vi "Insight_R_Synch_Index.vi"(8 "error in (no error)":errorcluster, 11 "telnet connection":T1) -> (0 "error out":errorcluster, 1 "response data":string, 2 "Index of Synch Pulse":u32, 3 "telnet  connection out":T1)   [LabVIEW 2015]
doc: "Insight Photonic Solutions\n\nThis VI reads the index of the Synchronization Pulse from the Synchronization sweep of the laser. Use this index, in comparison with a detected and acquired pulse, to synchronization the sweep with the acquisition.\n\nver 1.0 - original release\nver 1.1 - added output for the response data buffer"
uses:
  Telnet Session.ctl
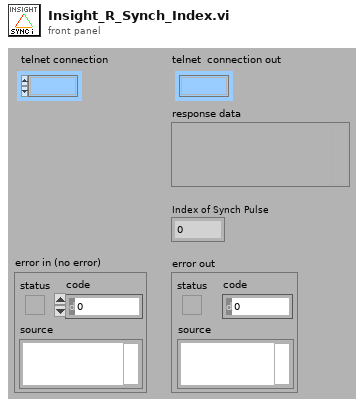
[diagram p1: front panel]
types:
  T1 = typedef "Telnet Session.ctl" = refnum<k1>
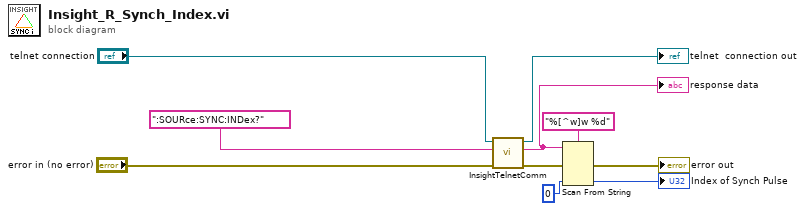
[diagram p0: block diagram]
diagram:
  n1 = call "InsightTelnetComm.vi"("error in"="error in (no error)", "write buffer (\"\")"=":SOURce:SYNC:INDex?" ("String"), "telnet connection"="telnet connection") -> ("error out"=w8:errorcluster, "response data"=w7:string, "telnet  connection out"=→"telnet  connection out":T1)  [unwired: 4 in]
  "response data" <- w7
  n2 = Scan From String(format string="%[^w]w %d", input string=w7, error in=w8, default 2=u32 0 ("default value 1")) -> (error out=→"error out":errorcluster, output 2=→"Index of Synch Pulse":u32)  [unwired: 3 in, 2 out]
